vi "Create.vi"(9 "Red Percent":dbl=10.0 format="%#_13g", 10 "Green Percent":dbl=5.0 format="%#_13g") -> (3 "Percent Difference out":refnum<class "Percent Difference.lvclass">)   [LabVIEW 2021, in "Percent Difference.lvclass"]
uses:
  Percent Difference.lvclass
  Percent Difference.lvclass/Percent Difference.ctl
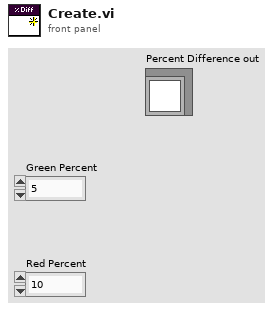
[diagram p1: front panel]
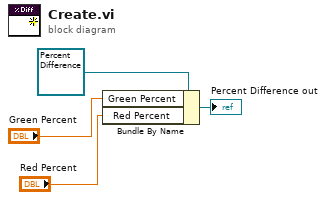
[diagram p0: block diagram]
diagram:
  n1 = Bundle By Name(cluster=refnum<class "Percent Difference.lvclass"> refnum ("Percent Difference in"), "Green Percent"="Green Percent", "Red Percent"="Red Percent") -> (→"Percent Difference out":refnum<class "Percent Difference.lvclass">)
